vi "INCLASS CONSTRUCTION.vi"() -> ()   [LabVIEW 2011]
panel:
  in  "stop":bool
  out "TEXT ALERT":string
  out "Enum":T1(ring)
  in  "START\nSWITCH":bool
  out "FEED TANK #2\n TEMPERATURE":dbl
  in  "FEED TANK  #2\nTEMP. CONTROL":dbl
  out "FEED TANK\n LEVEL #2":dbl
  in  "FEED TANK #2 \nLEVEL CONTROL":dbl
  out "FEED TANK \nLEVEL #1":dbl
  in  "FEED TANK #1\nLEVEL CONTROL":dbl
  out "MAIN TANK LEVEL":dbl
  in  "MAIN TANK \nLEVEL CONTROL":dbl
  in  "CONVEYOR\nPOSITION #2":bool
  in  "CONVEYOR\nPOSITION #1":bool
  out "HEATER":bool
  out "CONVEYOR":bool
  out "PUMP":bool
  out "DRAIN VALVE #2":bool
  out "DRAIN VALVE #1":bool
  out "FILL VALVE #2":bool
  out "FILL VALVE #1":bool
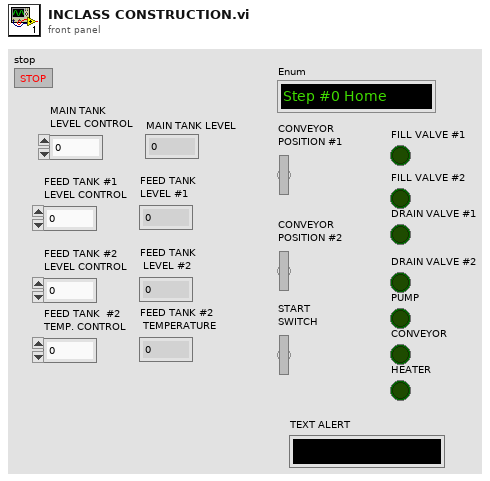
[diagram p1: front panel]
types:
  T1 = enum16{"Step #0 Home", "Step #1 Start System", "Step #2 Fill Tanks", "Step #3 Position #1", "Step #4 Fill #1", "Step #5 Position #2", "Step #6 Temperature", "Step #7 Fill #2"}
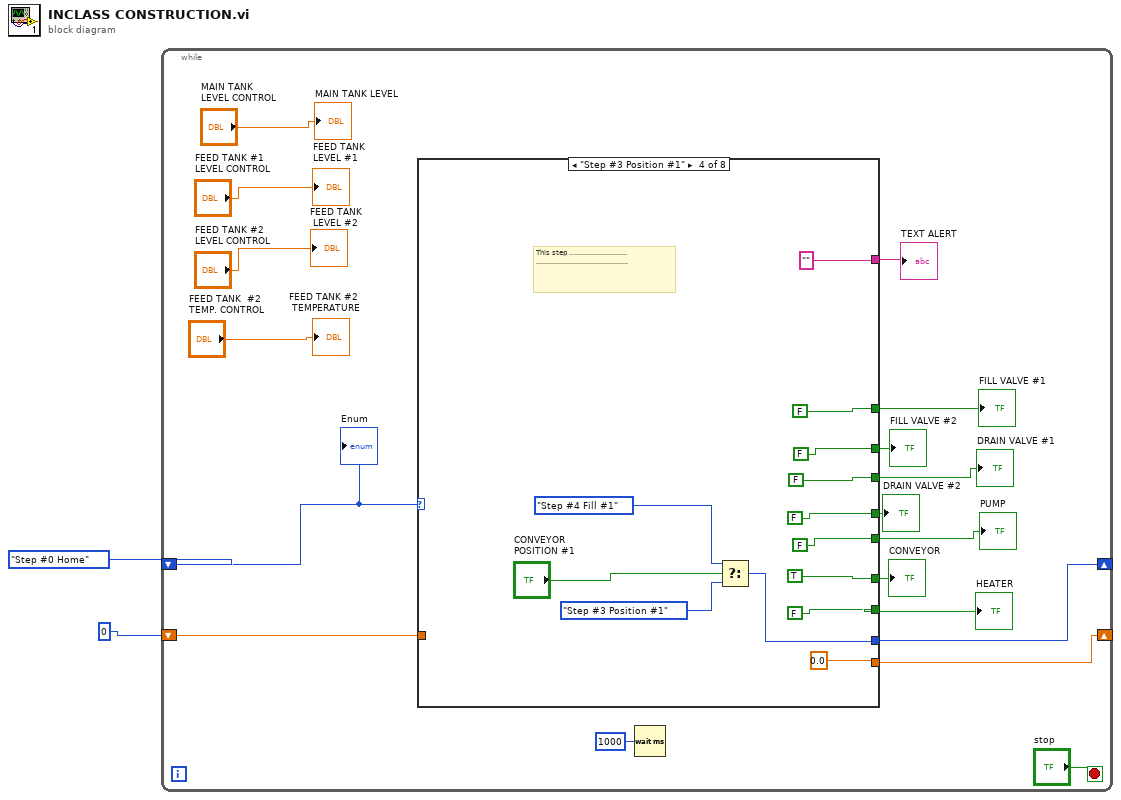
[diagram p0: block diagram]
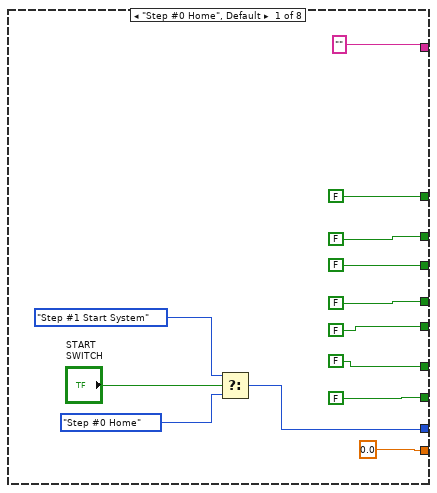
[diagram p2: hidden frame]
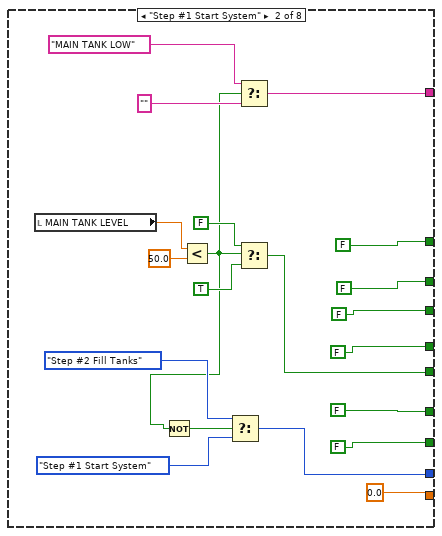
[diagram p3: hidden frame]
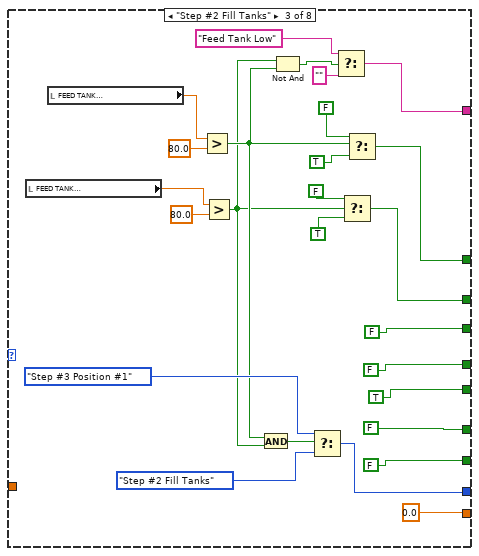
[diagram p4: hidden frame]
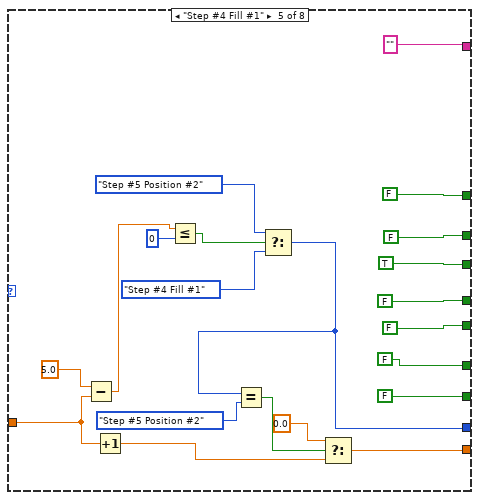
[diagram p5: hidden frame]
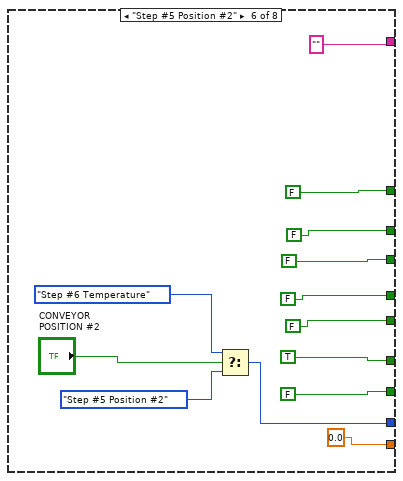
[diagram p6: hidden frame]
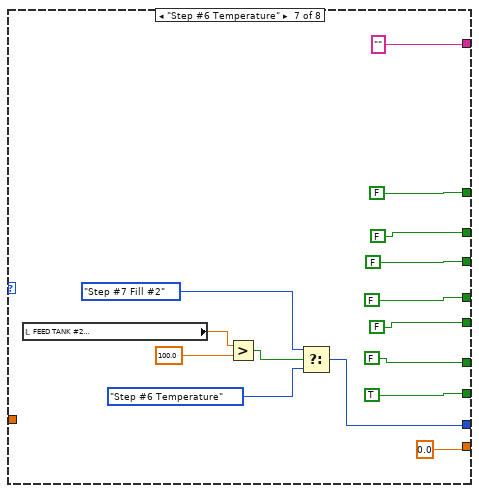
[diagram p7: hidden frame]
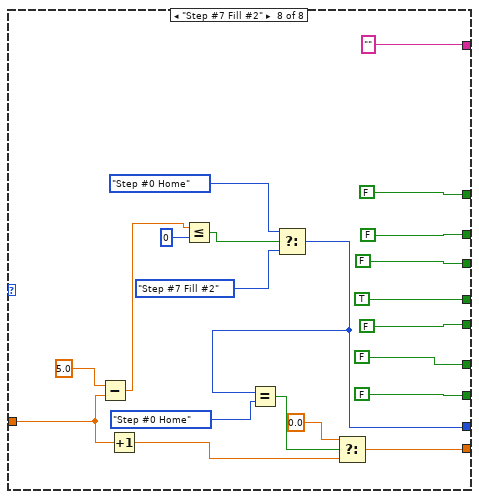
[diagram p8: hidden frame]
diagram:
  n1 = while {
    shift-right: [w12] -> _
    shift-left: T1."Step #0 Home" -> [w20]
    shift-right: [w5] -> _
    shift-left: 0 -> [w6]
    stop <- "stop" stop-if-true
    n2 = case shown="\"Step #3 Position #1\"" w20 {
      tunnel: [FALSE FALSE w62 FALSE FALSE FALSE FALSE FALSE] -> w19
      tunnel: [FALSE FALSE FALSE FALSE FALSE FALSE FALSE TRUE] -> w18
      tunnel: [FALSE FALSE w63 FALSE FALSE FALSE FALSE FALSE] -> w17
      tunnel: [FALSE FALSE FALSE TRUE FALSE TRUE FALSE FALSE] -> w16
      tunnel: [FALSE FALSE FALSE FALSE FALSE FALSE TRUE FALSE] -> w15
      tunnel: [FALSE FALSE FALSE FALSE TRUE FALSE FALSE FALSE] -> w14
      tunnel: [FALSE w42 TRUE FALSE FALSE FALSE FALSE FALSE] -> w13
      tunnel: [w24 w45 w72 w83 w94 w117 w132 w142] -> w12
      tunnel: ["" w35 w55 "" "" "" "" ""] -> w7
      tunnel: w6 -> [_ _ _ _ w98 _ _ w144]
      tunnel: [0.0 ("t") 0.0 ("t") 0.0 ("t") 0.0 ("t") w95 0.0 ("t") 0.0 ("t") w143] -> w5
      frame "Step #0 Home", Default {
        n3 = Select(t=T1."Step #1 Start System", s="START\nSWITCH", f=T1."Step #0 Home") -> (s? t:f=w24:T1)
      }
      frame "Step #1 Start System" {
        n4 = local read "MAIN TANK LEVEL"() -> (w43:dbl)
        n5 = Less?(x=w43, y=50.0) -> (x < y?=w36:bool)
        n6 = Not(x=w36) -> (.not. x?=w39:bool)
        n7 = Select(t=T1."Step #2 Fill Tanks", s=w39, f=T1."Step #1 Start System") -> (s? t:f=w45:T1)
        n8 = Select(t="MAIN TANK LOW", s=w36, f="") -> (s? t:f=w35:string)
        n9 = Select(t=FALSE, s=w36, f=TRUE) -> (s? t:f=w42:bool)
      }
      frame "Step #2 Fill Tanks" {
        n10 = local read "FEED TANK\n LEVEL #2"() -> (w69:dbl)
        n11 = local read "FEED TANK \nLEVEL #1"() -> (w68:dbl)
        n12 = Greater?(x=w68, y=80.0) -> (0:w57:bool)
        n13 = Greater?(x=w69, y=80.0) -> (0:w56:bool)
        n14 = And(x=w57, y=w56) -> (x .and. y?=w61:bool)
        n15 = Not And(1:w57, 2:w56) -> (0:w60:bool)
        n16 = Select(t=T1."Step #3 Position #1", s=w61, f=T1."Step #2 Fill Tanks") -> (s? t:f=w72:T1)
        n17 = Select(t="Feed Tank Low", s=w60, f="") -> (s? t:f=w55:string)
        n18 = Select(t=FALSE, s=w56, f=TRUE) -> (s? t:f=w62:bool)
        n19 = Select(t=FALSE, s=w57, f=TRUE) -> (s? t:f=w63:bool)
      }
      frame "Step #3 Position #1" {
        # "This step .............................\n.............................................."
        n20 = Select(t=T1."Step #4 Fill #1", s="CONVEYOR\nPOSITION #1", f=T1."Step #3 Position #1") -> (s? t:f=w83:T1)
      }
      frame "Step #4 Fill #1" {
        n21 = Subtract(x=5.0, y=w98) -> (x-y=w101:dbl)
        n22 = Increment(x=w98) -> (x+1=w99:dbl)
        n23 = Less Or Equal?(x=w101, y=u32 0) -> (x <= y?=w97:bool)
        n24 = Select(t=T1."Step #5 Position #2", s=w97, f=T1."Step #4 Fill #1") -> (s? t:f=w94:T1)
        n25 = Equal?(x=w94, y=T1."Step #5 Position #2") -> (x = y?=w96:bool)
        n26 = Select(t=0.0, s=w96, f=w99) -> (s? t:f=w95:dbl)
      }
      frame "Step #5 Position #2" {
        n27 = Select(t=T1."Step #6 Temperature", s="CONVEYOR\nPOSITION #2", f=T1."Step #5 Position #2") -> (s? t:f=w117:T1)
      }
      frame "Step #6 Temperature" {
        n28 = local read "FEED TANK #2\n TEMPERATURE"() -> (w127:dbl)
        n29 = Greater?(x=w127, y=100.0) -> (0:w129:bool)
        n30 = Select(t=T1."Step #7 Fill #2", s=w129, f=T1."Step #6 Temperature") -> (s? t:f=w132:T1)
      }
      frame "Step #7 Fill #2" {
        n31 = Subtract(x=5.0, y=w144) -> (x-y=w150:dbl)
        n32 = Increment(x=w144) -> (x+1=w148:dbl)
        n33 = Less Or Equal?(x=w150, y=u32 0) -> (x <= y?=w147:bool)
        n34 = Select(t=T1."Step #0 Home", s=w147, f=T1."Step #7 Fill #2") -> (s? t:f=w142:T1)
        n35 = Equal?(x=w142, y=T1."Step #0 Home") -> (x = y?=w146:bool)
        n36 = Select(t=0.0, s=w146, f=w148) -> (s? t:f=w143:dbl)
      }
    }
    "FILL VALVE #2" <- w19
    "DRAIN VALVE #1" <- w14
    "HEATER" <- w15
    "CONVEYOR" <- w16
    "FILL VALVE #1" <- w17
    "DRAIN VALVE #2" <- w18
    "PUMP" <- w13
    "TEXT ALERT" <- w7
    n37 = Wait (ms)(milliseconds to wait=u32 1000) -> ()  [unwired: 1 out]
    "Enum" <- w20
    "FEED TANK #2\n TEMPERATURE" <- "FEED TANK  #2\nTEMP. CONTROL"
    "FEED TANK \nLEVEL #1" <- "FEED TANK #1\nLEVEL CONTROL"
    "MAIN TANK LEVEL" <- "MAIN TANK \nLEVEL CONTROL"
    "FEED TANK\n LEVEL #2" <- "FEED TANK #2 \nLEVEL CONTROL"
  }
